vi "ex_Caesar Cypher.vi"() -> ()   [LabVIEW 2015]
uses:
  Letter/Letter.lvclass
  objdict/objdict.lvclass
panel:
  out "Encrypted Text (Variant attribute dict)":string
  out "Encrypted Text (objdict)":string
  in  "Enter Text to encrypt":string
  in  "Shift":u8=11
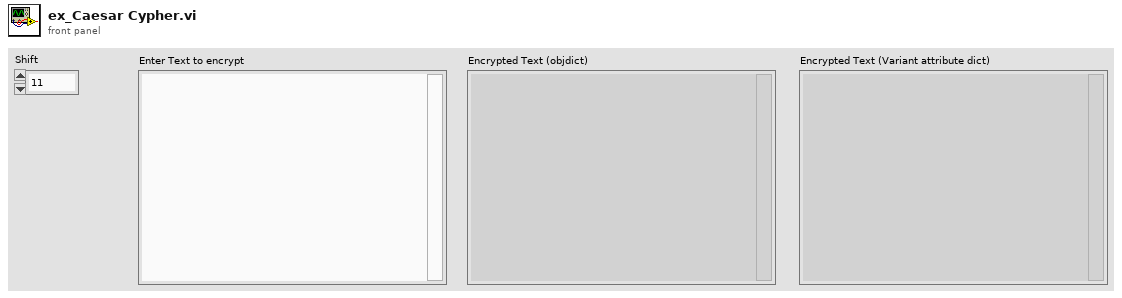
[diagram p1: front panel]
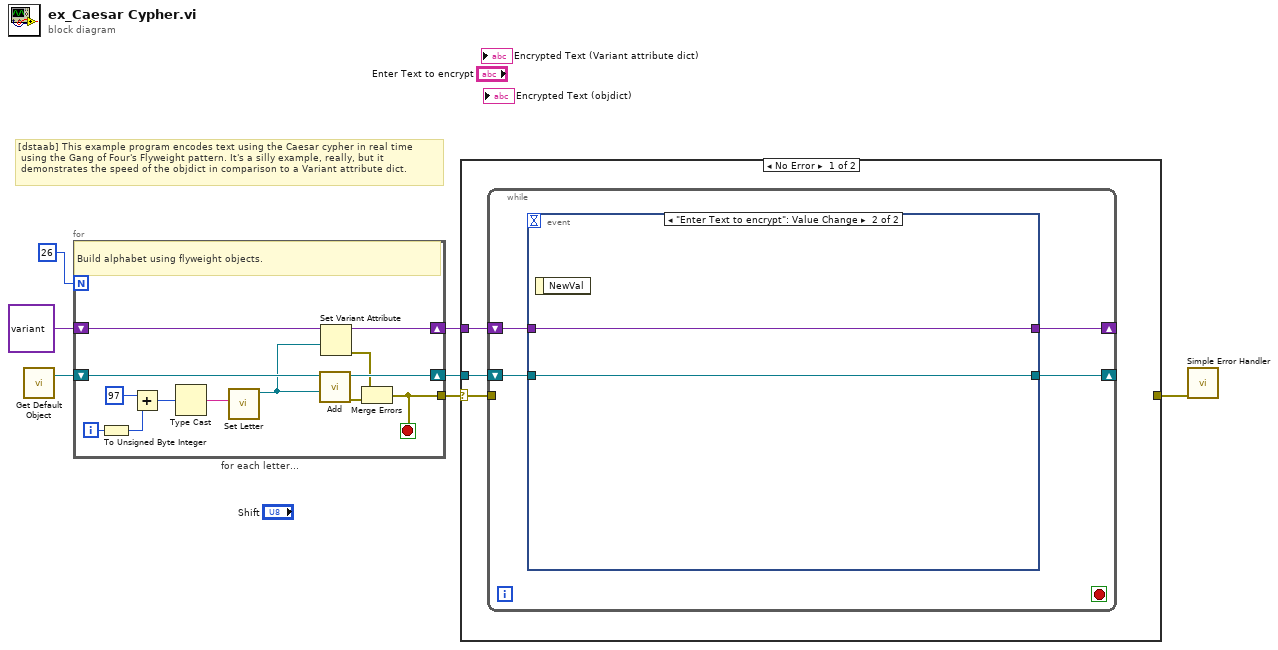
[diagram p0: block diagram]
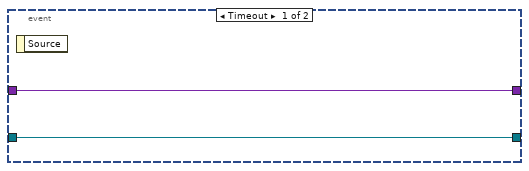
[diagram p2: hidden frame]
diagram:
  # "[dstaab] This example program encodes text using the Caesar cypher in real time\n using the Gang of Four's Flyweight pattern. It's a silly example, really, but it\n demonstrates the speed of the objdict in comparison to a Variant attribute dict."
  n1 = call "Get Default Object.vi"() -> ("Object Dictionary"=w6:refnum<class "objdict.lvclass">)  [unwired: 1 in]
  n2 = for "for each letter..." {
    N: 26 -> [_]
    shift-right: [w17] -> w1
    shift-left: w6 -> [w16]
    shift-right: [w13] -> w2
    shift-left: variant -> [w12]
    tunnel: [w8] -> w4
    i -> [w20]
    stop <- w8 stop-if-true
    # "Build alphabet using flyweight objects."
    n3 = To Unsigned Byte Integer(number=w20) -> (unsigned 8bit integer=w14:u8)
    n4 = Add(x=u8 97, y=w14) -> (x+y=w15:u8)
    n5 = Type Cast(x=w15) -> (*(type *) &x=w18:string)  [unwired: 1 in]
    n6 = call "Set Letter.vi"("letter"=w18) -> ("Letter out"=w11:refnum<class "Letter.lvclass">)  [unwired: 10 in]
    n7 = call "Add.vi"("LabVIEW Object"=w11, "Object Dictionary in (new)"=w16) -> ("error out"=w10:errorcluster, "Object Dictionary out"=w17:refnum<class "objdict.lvclass">)  [unwired: 8 in]
    n8 = Set Variant Attribute(Variant=w12, value=w11) -> (Variant out=w13:variant, error out=w9:errorcluster)  [unwired: 2 in, 1 out]
    n9 = Merge Errors(w9, w10) -> (w8:errorcluster)
  }
  n10 = case shown="No Error" w4 {
    selector: w4 -> [w23 w32]
    tunnel: [_ w32] -> w3
    tunnel: w2 -> [w22 _]
    tunnel: w1 -> [w21 _]
    frame No Error {
      n11 = while {
        tunnel: w23 -> [_]
        shift-right: [w25] -> _
        shift-left: w22 -> [w27]
        shift-right: [w24] -> _
        shift-left: w21 -> [w26]
        stop <- _ stop-if-true
        n12 = event shown="[1] \"Enter Text to encrypt\": Value Change" {
          selector: _ -> [_ _]
          dyn-events: _ -> [_ _]
          timeout: _ -> [_ _]
          tunnel: w27 -> [w29 w31]
          tunnel: w26 -> [w28 w30]
          tunnel: [w29 w31] -> w25
          tunnel: [w28 w30] -> w24
          event Timeout {
            n13 = event-data() -> ()  [unwired: 1 in, 1 out]
          }
          event "Enter Text to encrypt": Value Change {
            n14 = event-data() -> ()  [unwired: 1 in, 1 out]
          }
        }
      }
    }
    frame Error {
    }
  }
  n15 = call <vilib>:"Simple Error Handler.vi"("error in (no error)"=w3) -> ()  [unwired: 4 in, 5 out]
